vi "Sort 1D Double.vi"(1 "1D input array":dbl[](array[numeric])) -> (0 "output array":dbl[](array[numeric]))   [LabVIEW 2018]
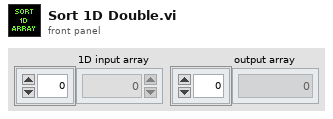
[diagram p1: front panel]
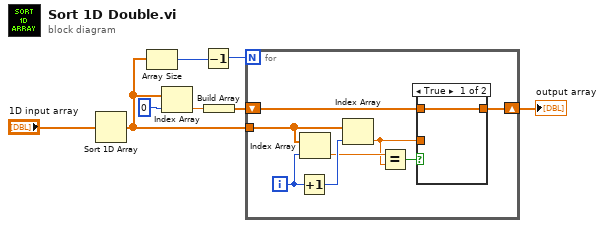
[diagram p0: block diagram]
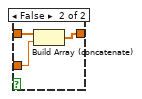
[diagram p2: hidden frame]
diagram:
  n1 = Sort 1D Array(array="1D input array") -> (sorted array=w5:dbl[])
  n2 = Array Size(array=w5) -> (size(s)=w8:i32)
  n3 = Index Array(array=w5, index=0) -> (element=w4:dbl)
  n4 = Decrement(x=w8) -> (x-1=w7:i32)
  n5 = Build Array(w4) -> (w3:dbl[])
  n6 = for {
    N: w7 -> [_]
    tunnel: w5 -> [w14]
    shift-right: [w11] -> w1
    shift-left: w3 -> [w12]
    i -> [w15]
    n7 = Increment(x=w15) -> (x+1=w16:i32)
    n8 = Index Array(array=w14, index=w15) -> (element=w10:dbl)
    n9 = Index Array(array=w14, index=w16) -> (element=w9:dbl)
    n10 = Equal?(x=w10, y=w9) -> (x = y?=w13:bool)
    n11 = case shown="True" w13 {
      tunnel: w9 -> [_ w20]
      tunnel: w12 -> [w17 w19]
      tunnel: [w17 w18] -> w11
      frame True {
      }
      frame False {
        n12 = Build Array (concatenate)(w19, w20) -> (w18:dbl[])
      }
    }
  }
  "output array" <- w1
